vi "Handle Knob Settings.vi"(6 "Table Setting Name in":string, 7 "Write? (F:Read)":bool, 8 "error in (no error)":errorcluster, 9 "Knob":refnum<vi>, 11 "Save Restore Settings in":refnum<class "Save Restore Settings.lvclass">) -> (0 "error out":errorcluster, 1 "Sub Controls":T1[](array[typedef]), 3 "Save Restore Settings out":refnum<class "Save Restore Settings.lvclass">)   [LabVIEW 2020, in "Save Restore Settings.lvclass"]
uses:
  <userlib>/_MGI/Application Control/MGI Save Restore Settings/Save Restore Settings.lvclass
  <userlib>/_MGI/Application Control/MGI Save Restore Settings/Control Info.ctl
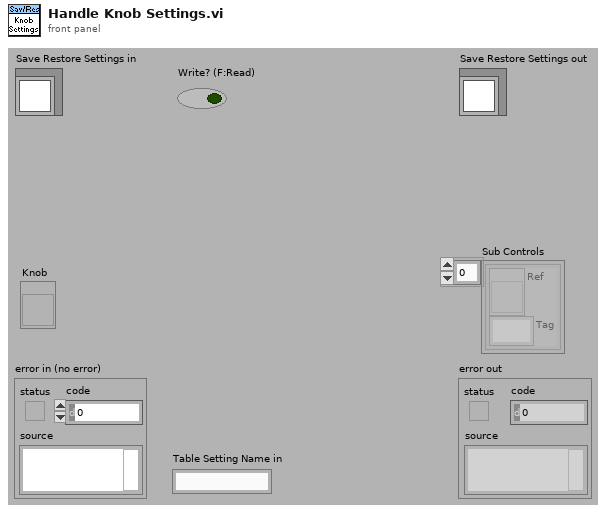
[diagram p1: front panel]
types:
  T1 = typedef "Save Restore Settings.lvclass/Control Info.ctl" = cluster{"Ref":refnum<vi>, "Tag":string}
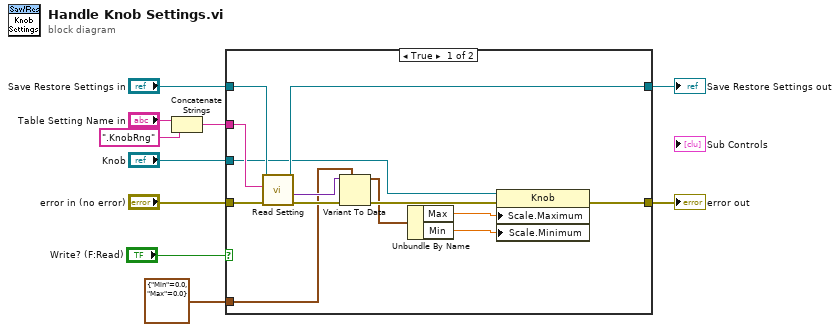
[diagram p0: block diagram]
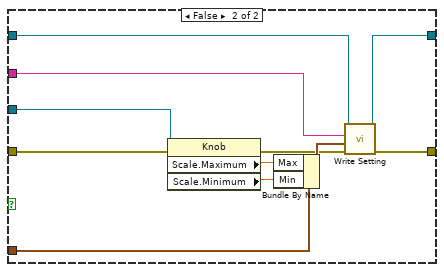
[diagram p2: hidden frame]
diagram:
  n1 = Concatenate Strings("Table Setting Name in", ".KnobRng" ("string")) -> (w3:string)
  n2 = case shown="True" "Write? (F:Read)" {
    tunnel: "Knob" -> [w16 w34]
    tunnel: "error in (no error)" -> [w21 w33]
    tunnel: "Save Restore Settings in" -> [w19 w27]
    tunnel: [w18 w26] -> w7
    tunnel: [w17 w24] -> w6
    tunnel: w3 -> [w20 w28]
    tunnel: cluster{"Min":dbl, "Max":dbl} {"Min"=0.0, "Max"=0.0} -> [w14 w32]
    frame True {
      n3 = call-dynamic "Read Setting.vi"("error in (no error)"=w21, "Tag Name"=w20, "Save Restore Settings in"=w19) -> ("error out"=w22:errorcluster, "Tag Attribute"=w23:variant, "Save Restore Settings out"=w18:refnum<class "Save Restore Settings.lvclass">)  [unwired: 6 in]
      n4 = Variant To Data(error in=w22, type=w14, Variant=w23) -> (data=w13:cluster{"Min":dbl, "Max":dbl}, error out=w15:errorcluster)
      n5 = Unbundle By Name(w13) -> ("Max"=w12:dbl, "Min"=w11:dbl)
      n6 = property class="Knob"(reference=w16, error in=w15, "Scale.Maximum"=w12, "Scale.Minimum"=w11) -> (error out=w17:errorcluster)  [unwired: 1 out]
    }
    frame False {
      n7 = property class="Knob"(reference=w34, error in=w33) -> (error out=w25:errorcluster, "Scale.Maximum"=w31:dbl, "Scale.Minimum"=w30:dbl)  [unwired: 1 out]
      n8 = Bundle By Name(cluster=w32, "Max"=w31, "Min"=w30) -> (w29:cluster{"Min":dbl, "Max":dbl})
      n9 = call-dynamic "Write Setting.vi"("error in (no error)"=w25, "Tag Attribute"=w29, "Tag Name"=w28, "Save Restore Settings in"=w27) -> ("error out"=w24:errorcluster, "Save Restore Settings out"=w26:refnum<class "Save Restore Settings.lvclass">)  [unwired: 6 in]
    }
  }
  "error out" <- w6
  "Save Restore Settings out" <- w7
